vi "stopAutomatedTest.vi"(8 "error in (no error)":errorcluster, 10 "model":refnum<class "Model.lvclass">, 11 "AutomatedMotionState in":refnum<class "AutomatedProfileState.lvclass">) -> (0 "error out":errorcluster, 2 "model 2":refnum<class "Model.lvclass">, 3 "AutomatedMotionState out":refnum<class "AutomatedProfileState.lvclass">)   [LabVIEW 2013, in "AutomatedProfileState.lvclass"]
uses:
  AutomatedProfileState.lvclass
  Model/Model/Model.lvclass
  Typedefs/StateSelector.ctl
  Typedefs/FAMTTypedefs.lvlib
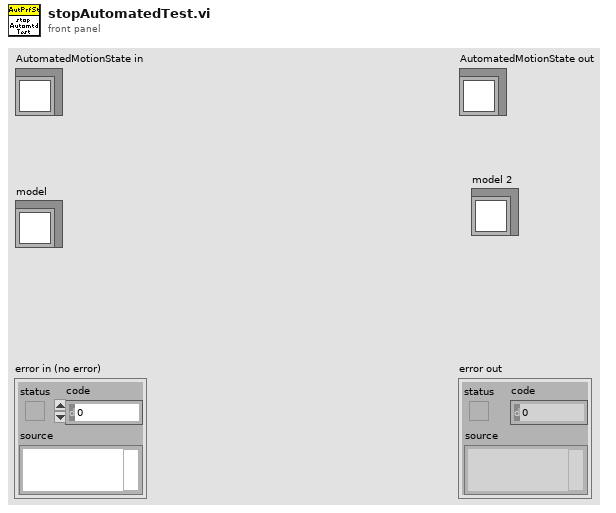
[diagram p1: front panel]
types:
  T1 = typedef "FAMTTypedefs.lvlib/StateSelector.ctl" = enum16{"EndingCycleState", "FaultState", "InteractiveSetpointState", "OffState", "StandbyState", "StoppedState"}
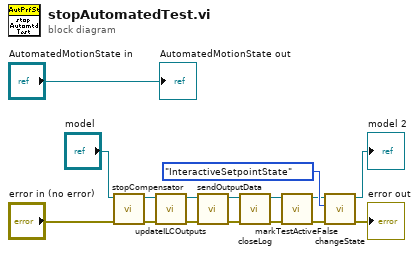
[diagram p0: block diagram]
diagram:
  n1 = call "stopCompensator.vi"("error in (no error)"="error in (no error)", "Model in"="model") -> ("error out"=w4:errorcluster, "Model out"=w6:refnum<class "Model.lvclass">)  [unwired: 8 in]
  n2 = call "updateILCOutputs.vi"("error in (no error)"=w4, "Model in"=w6) -> ("error out"=w3:errorcluster, "Model out"=w5:refnum<class "Model.lvclass">)  [unwired: 8 in]
  n3 = call "sendOutputData.vi"("error in (no error)"=w3, "Model in"=w5) -> ("error out"=w1:errorcluster, "Model out"=w2:refnum<class "Model.lvclass">)  [unwired: 8 in]
  n4 = call "closeLog.vi"("error in (no error)"=w1, "Model in"=w2) -> ("error out"=w7:errorcluster, "Model out"=w8:refnum<class "Model.lvclass">)  [unwired: 8 in]
  n5 = call "markTestActiveFalse.vi"("error in (no error)"=w7, "Model in"=w8) -> ("error out"=w9:errorcluster, "Model out"=w10:refnum<class "Model.lvclass">)  [unwired: 8 in]
  n6 = call "changeState.vi"("error in (no error)"=w9, "State:"=StateSelector."InteractiveSetpointState", "Model in"=w10) -> ("error out"=→"error out":errorcluster, "Model out"=→"model 2":refnum<class "Model.lvclass">)  [unwired: 7 in]
  "AutomatedMotionState out" <- "AutomatedMotionState in"
